vi "Dynamic Control Position (Tab).vi"(4 "Top Offset (%)":dbl, 6 "Left Offset (%)":dbl, 7 "Control Ref":refnum<vi>, 8 "error in (no error)":errorcluster, 9 "Position":T1, 10 "Width(%)":dbl, 11 "Height(%)":dbl) -> (0 "error out":errorcluster, 1 "Start Pos of next control":T1)   [LabVIEW 2014]
uses:
  <vilib>/Utility/miscctls.llb/LVPositionTypeDef.ctl
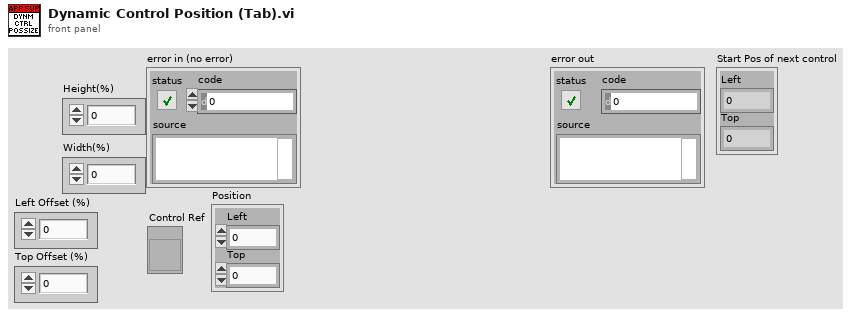
[diagram p1: front panel]
types:
  T1 = typedef "LVPositionTypeDef.ctl" = cluster{"Left":i32, "Top":i32}
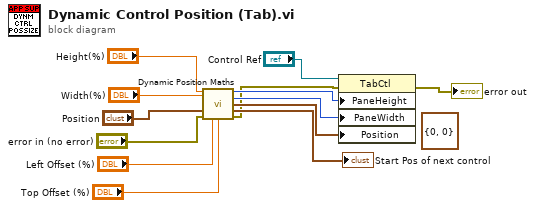
[diagram p0: block diagram]
diagram:
  (unwired) T1 {"Left"=0, "Top"=0} ("Position")
  n1 = call "Dynamic Position Maths.vi"("Height(%)"="Height(%)", "Width(%)"="Width(%)", "Position"="Position", "error in (no error)"="error in (no error)", "Left Offset (%)"="Left Offset (%)", "Top Offset (%)"="Top Offset (%)") -> ("Height"=w8:u32, "Width"=w7:u32, "Position Out"=w6:T1, "Start Pos of next control"=→"Start Pos of next control":T1, "error out"=w4:errorcluster)  [unwired: 5 in]
  n2 = property class="TabCtl"(reference="Control Ref", error in=w4, "PaneHeight"=w8, "PaneWidth"=w7, "Position"=w6) -> (error out=→"error out":errorcluster)  [unwired: 1 out]
